vi "Test - Calculate Projection Matrix.vi"   [LabVIEW 2022 SP3, in "3D.lvlib"]
uses:
  3D.lvlib
  Raster/Screen Dimensions.ctl
  Camera.ctl
  Calculate A F Q.vi
  Degrees To Radians.vi
  <vilib>/addons/_JKI Toolkits/Caraya/classes/Assert/Assert Equal Value and Type_Variant.vi
  Raster/Raster.lvlib
  <vilib>/addons/_JKI Toolkits/Caraya/classes/Test/Test.lvclass
  <vilib>/addons/_JKI Toolkits/Caraya/classes/Assert/Assert.lvclass
types:
  T1 = typedef "3D.lvlib/Camera.ctl" = cluster{"Field Of View":sgl, "Near Plane":sgl, "Far Plane":sgl}
  T2 = typedef "Raster.lvlib/Screen Dimensions.ctl" = cluster{"Width":u32, "Height":u32}
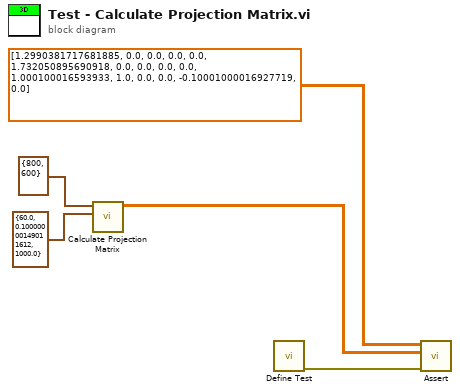
[diagram p0: block diagram]
diagram:
  n1 = call "Calculate Projection Matrix.vi"("Camera"=T1 {"Field Of View"=60.0, "Near Plane"=0.1, "Far Plane"=1000.0}, "Screen Dimensions"=T2 {"Width"=800, "Height"=600}) -> ("Projection Matrix"=w2:sgl[][])  [unwired: 9 in]
  n2 = call <vilib>:"Define Test.vi"() -> ("error out"=w1:errorcluster)  [unwired: 11 in]
  n3 = call-poly <vilib>:"Assert.vi"("error in (no error)"=w1, "Y"=w2, "X"=sgl[][] [[1.2990382, 0.0, 0.0, 0.0], [0.0, 1.7320509, 0.0, 0.0], [0.0, 0.0, 1.0001, 1.0], [0.0, 0.0, -0.10001, 0.0]] ("Projection Matrix")) -> ()  [unwired: 8 in, 1 out]
